vi "Convert string of numbers to array.vi"(4 "delimiter (Coma)":string=",", 5 "#'s string":string="1-4") -> (2 "#'s Array":i16[](array[numeric]))   [LabVIEW 2015]
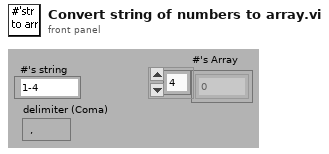
[diagram p1: front panel]
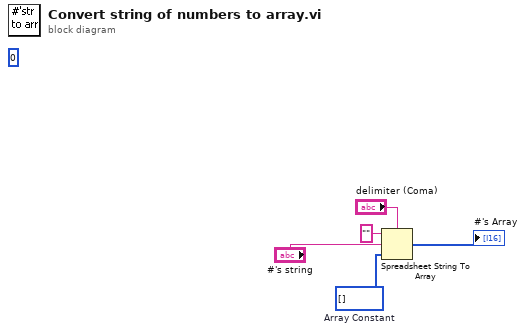
[diagram p0: block diagram]
diagram:
  w5 = i16[] []  # Array Constant
  (unwired) 0
  n1 = Spreadsheet String To Array(delimiter (Tab)="delimiter (Coma)", format string="", spreadsheet string="#'s string", array type (2D Dbl)=w5) -> (array=→"#'s Array":i16[])
